vi "Destroy.vi"(11 "Base Queue in":refnum<class "Base Queue.lvclass">) -> (3 "Base Queue out":refnum<class "Base Queue.lvclass">)   [LabVIEW 2021, in "jettl.lvlib" / "Base Queue.lvlib" / "Base Queue.lvclass"]
uses:
  Base Queue.lvclass
  Base Queue.lvclass/Base Queue.ctl
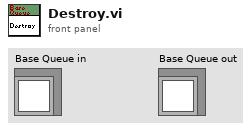
[diagram p1: front panel]
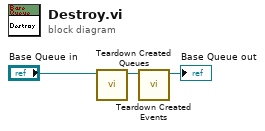
[diagram p0: block diagram]
diagram:
  n1 = call-dynamic "Teardown Created Queues.vi"("Base Queue in"="Base Queue in") -> ("Base Queue out"=w3:refnum<class "Base Queue.lvclass">)  [unwired: 10 in]
  n2 = call-dynamic "Teardown Created Events.vi"("Base Queue in"=w3) -> ("Base Queue out"=→"Base Queue out":refnum<class "Base Queue.lvclass">)  [unwired: 10 in]
